vi "DSF.Engine.Plugin.Get Debug Flags.vi"(11 "Plugin in":refnum<class "DSF.Engine.Plugin.lvclass">) -> (2 "Debug Flags":refnum<class "DSF.Engine.Debug Flags.lvclass">, 3 "Plugin out":refnum<class "DSF.Engine.Plugin.lvclass">)   [LabVIEW 2017, in "Data Sharing Framework Engine.lvlib" / "DSF.Engine.Plugin.lvclass"]
uses:
  DSF.Engine.Plugin.lvclass
  Debug/DSF.Engine.Debug Flags.lvclass
  DSF.Engine.Plugin.lvclass/DSF.Engine.Plugin.ctl
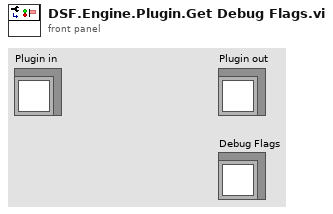
[diagram p1: front panel]
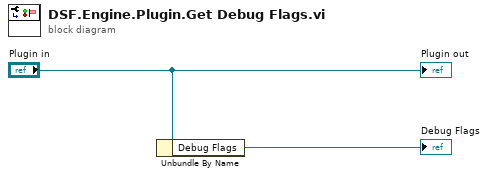
[diagram p0: block diagram]
diagram:
  n1 = Unbundle By Name("Plugin in") -> ("Debug Flags"=→"Debug Flags":refnum<class "DSF.Engine.Debug Flags.lvclass">)
  "Plugin out" <- "Plugin in"
